vi "Get Aperture Time Info [DT].vi"(8 "error in (no error)":errorcluster, 11 "CS++DMM in":refnum<class "CS++DMM.lvclass">) -> (0 "error out":errorcluster, 1 "aperture time units":i32, 2 "aperture time (sec)":dbl format="%^.2e", 3 "CS++DMM out":refnum<class "CS++DMM.lvclass">)   [LabVIEW 2013, in "CS++DMM.lvlib" / "CS++DMM.lvclass"]
doc: "This VI returns additional information about the state of the instrument. Specifically, it returns the aperture time and the aperture time units.\n\nNote: \n\n(1) This VI is part of the IviDmmDeviceInfo [DI] extension group."
uses:
  CS++DMM.lvclass
  CSPP_Core/Classes/CS++ProcessVariables/ProcessVariable/PV.lvclass
  CSPP_Core/Classes/CS++ProcessVariables/ProcessVariable/PV.lvclass/PV.ctl
  CS++DMM.lvclass/CS++DMM.ctl
  CSPP_Core/Classes/CS++ProcessVariables/PVConnection/PVConnection.lvclass
  CSPP_Core/Classes/CS++ProcessVariables/ProcessVariable/Write Data.vi
  CSPP_Core/Classes/CS++ProcessVariables/ProcessVariable/Write Timestamp.vi
  CSPP_Core/Classes/CS++ProcessVariables/ProcessVariable/Write Quality.vi
  CSPP_Core/Classes/CS++ProcessVariables/ProcessVariable/Write status.vi
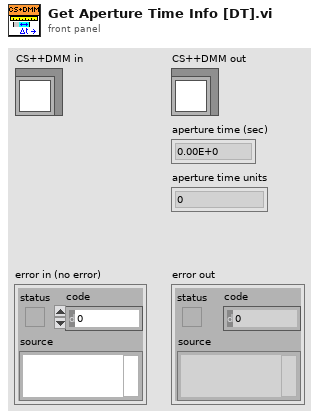
[diagram p1: front panel]
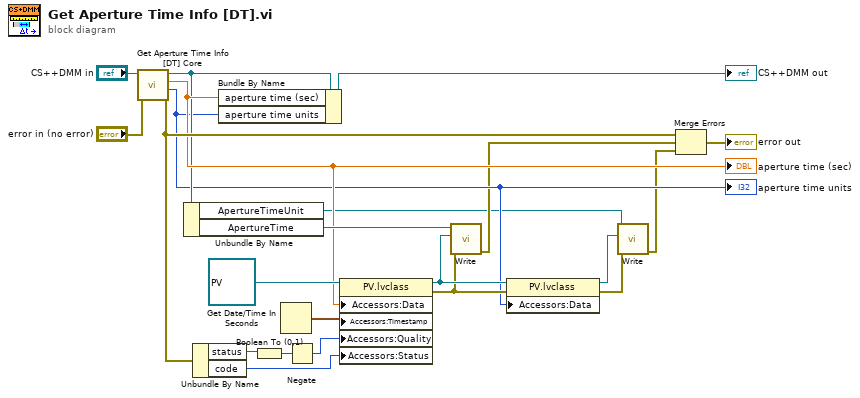
[diagram p0: block diagram]
diagram:
  n1 = call-dynamic "Get Aperture Time Info [DT] Core.vi"("error in (no error)"="error in (no error)", "CS++DMM in"="CS++DMM in") -> ("error out"=w13:errorcluster, "aperture time units"=w6:i32, "aperture time (sec)"=w12:dbl, "CS++DMM out"=w11:refnum<class "CS++DMM.lvclass">)  [unwired: 6 in]
  "aperture time (sec)" <- w12
  "aperture time units" <- w6
  n2 = Unbundle By Name(w11) -> ("ApertureTimeUnit"=w1:refnum<class "PVConnection.lvclass">, "ApertureTime"=w20:refnum<class "PVConnection.lvclass">)
  n3 = Unbundle By Name(w13) -> ("status"=w18:bool, "code"=w15:i32)
  n4 = Bundle By Name(cluster=w11, "aperture time (sec)"=w12, "aperture time units"=w6) -> (→"CS++DMM out":refnum<class "CS++DMM.lvclass">)
  n5 = Boolean To (0,1)(Boolean=w18) -> (0, 1=w17:i16)
  n6 = Get Date/Time In Seconds() -> (seconds since 1Jan1904=w14:timestamp)
  n7 = Negate(x=w17) -> (-x=w16:i16)
  n8 = property class="PV.lvclass"(reference=refnum<class "PV.lvclass"> refnum ("CS++ProcessVariables.lvlib:PV.lvclass"), "Accessors:Data"=w12, "Accessors:Timestamp"=w14, "Accessors:Quality"=w16, "Accessors:Status"=w15) -> (reference out=w8:refnum<class "PV.lvclass">, error out=w7:errorcluster)  [unwired: 1 in]
  n9 = call-dynamic "Write.vi"("error in (no error)"=w7, "PV"=w8, "PVConnection in"=w20) -> ("error out"=w3:errorcluster)  [unwired: 7 in, 1 out]
  n10 = property class="PV.lvclass"(reference=w8, error in=w7, "Accessors:Data"=w6) -> (reference out=w9:refnum<class "PV.lvclass">, error out=w5:errorcluster)
  n11 = call-dynamic "Write.vi"("error in (no error)"=w5, "PV"=w9, "PVConnection in"=w1) -> ("error out"=w2:errorcluster)  [unwired: 7 in, 1 out]
  n12 = Merge Errors(w13, w3, w2) -> (→"error out":errorcluster)
